vi "Create SFTP Refnum.vi"(8 "error in (no error)":errorcluster, 11 "LIBSSH2_SFTP*":u64 format="%.0x") -> (0 "error out":errorcluster, 3 "sftp":T1)   [LabVIEW 2013, in "libssh2.lvlib"]
doc: "Create SFTP refnum for <B>LIBSSH2_SFTP*</B>."
uses:
  libssh2.lvlib
  SFTP Refnum.ctl
  SFTP Refnum Data.ctl
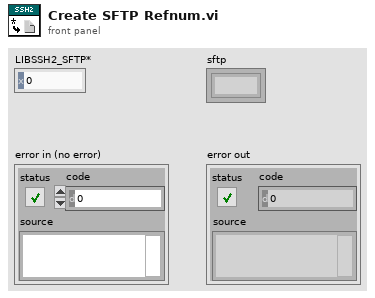
[diagram p1: front panel]
types:
  T1 = typedef "libssh2.lvlib/SFTP Refnum.ctl" = refnum<k1>
  T2 = typedef "libssh2.lvlib/SFTP Refnum Data.ctl" = cluster{"LIBSSH2_SFTP*":u64}
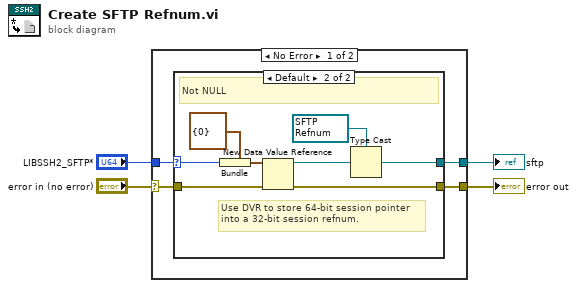
[diagram p0: block diagram]
diagram:
  n1 = case shown="No Error" "error in (no error)" {
    selector: "error in (no error)" -> [w6 w18]
    tunnel: [w8 _] -> w4
    tunnel: [w7 w18] -> w3
    tunnel: "LIBSSH2_SFTP*" -> [w5 _]
    frame No Error {
      n2 = case shown="Default" w5 {
        selector: w5 -> [_ w15]
        tunnel: [_ w16] -> w8
        tunnel: [w9 w13] -> w7
        tunnel: w6 -> [w9 w12]
        frame 0 {
          # "NULL"
        }
        frame Default {
          w17 = T1 refnum items=["sftp"] ("sftp")
          # "Use DVR to store 64-bit session pointer\ninto a 32-bit session refnum."
          # "Not NULL"
          n3 = Bundle(cluster=T2 {"LIBSSH2_SFTP*"=0} ("sftp data"), "LIBSSH2_SFTP*"=w15) -> (w11:T2)
          n4 = New Data Value Reference(data value=w11, error in=w12) -> (data value reference=w14:refnum<data-value>, error out=w13:errorcluster)
          n5 = Type Cast(type=w17, x=w14) -> (*(type *) &x=w16:T1)
        }
      }
    }
    frame Error {
    }
  }
  "sftp" <- w4
  "error out" <- w3
